vi "QTMTask.vi"(5 "timeout ms (25000)":i32=25000, 6 "Stop":bool, 7 "error in":errorcluster, 8 "ArrayIn":dbl[](array[numeric]), 9 "QTMqueue":refnum<queue>, 10 "connection ID":refnum<k5>) -> (0 "error out":errorcluster, 3 "connection ID out":refnum<k5>)   [LabVIEW 2010]
panel:
  out "ArrayOut":dbl[](array[numeric])
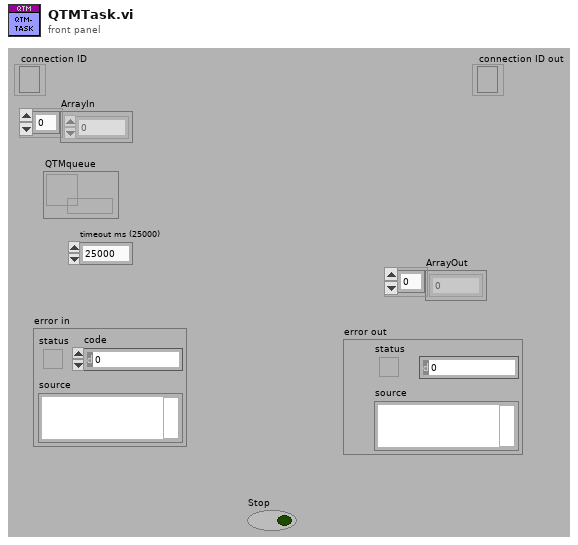
[diagram p1: front panel]
types:
  T1 = typedef "QTM Data Frame.ctl" = cluster{"Timestamp":i64, "Framenumber":i32, "ComponentCount":i32, "Components":cluster{"ComponentSize":i32, "ComponentType":T2, "Count":i32, "Padding":i32, "Data":dbl[][]}[]}
  T2 = typedef "QTM ComonentType.ctl" = i32
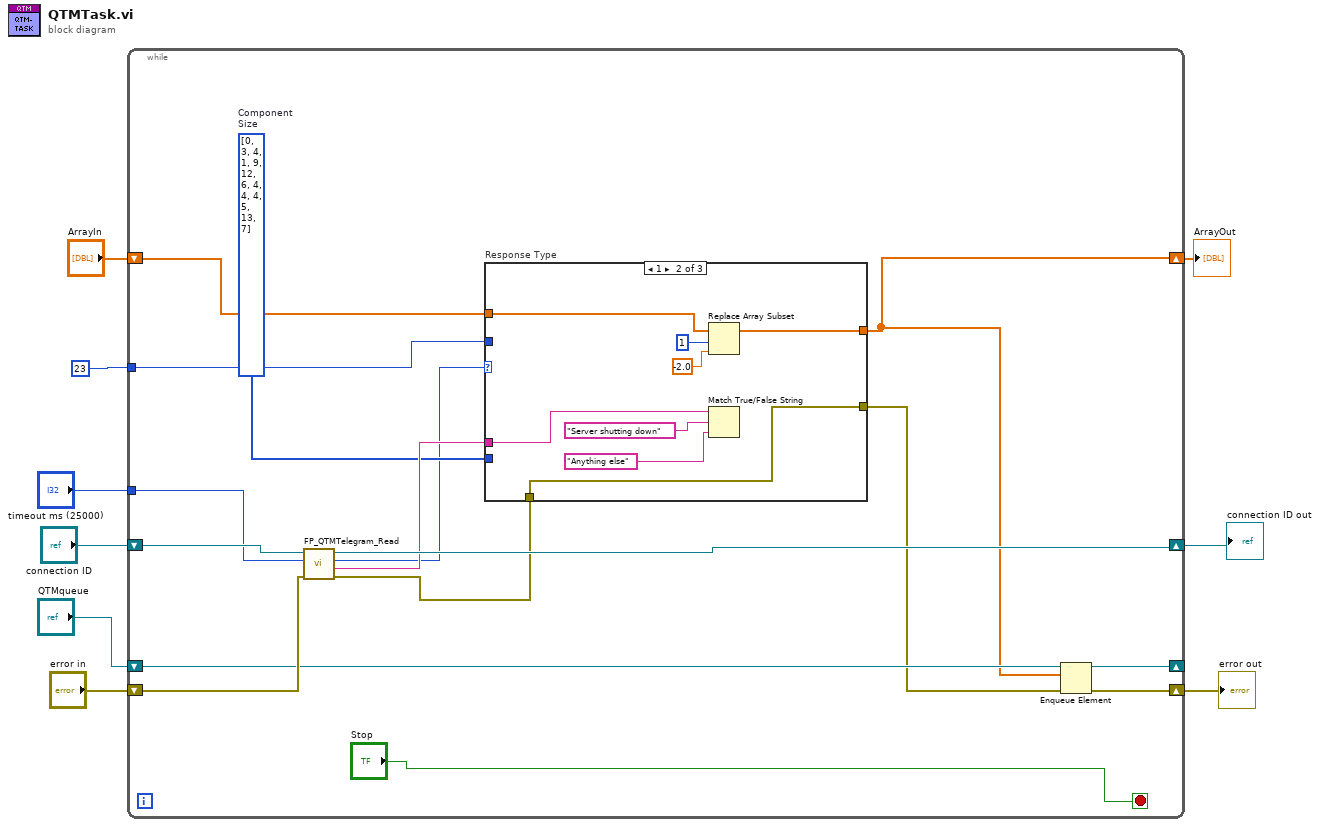
[diagram p0: block diagram]
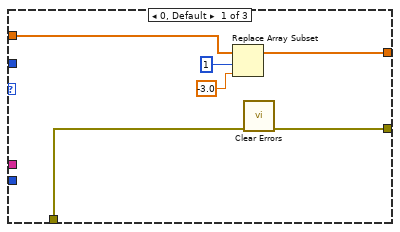
[diagram p2: hidden frame]
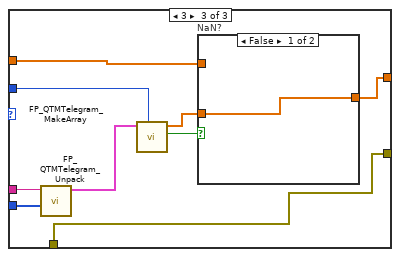
[diagram p3: hidden frame]
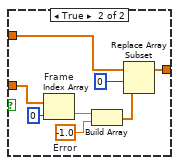
[diagram p4: hidden frame]
diagram:
  n1 = while {
    shift-right: [w12] -> w4
    shift-left: "ArrayIn" -> [w25]
    tunnel: 23 -> [w24]
    shift-right: [w13] -> w8
    shift-left: "error in" -> [w23]
    shift-right: [w21] -> w6
    shift-left: "connection ID" -> [w22]
    tunnel: "timeout ms (25000)" -> [w20]
    shift-right: [w15] -> _
    shift-left: "QTMqueue" -> [w16]
    stop <- "Stop" stop-if-true
    w18 = i32[] [0, 3, 4, 1, 9, 12, 6, 4, 4, 4, 5, 13, 7]  # Component Size
    n2 = call "FP_QTMTelegram_Read.vi"("error in (no error)"=w23, "timeout ms (25000)"=w20, "connection ID in"=w22) -> ("error out"=w14:errorcluster, "Data"=w19:string, "Response type"=w17:i32, "connection ID out"=w21:refnum<k5>)  [unwired: 5 out]
    n3 = case "Response Type" shown="1" w17 {
      tunnel: w19 -> [_ w37 w48]
      tunnel: [w30 w34 w45] -> w12
      tunnel: w18 -> [_ _ w43]
      tunnel: w24 -> [_ _ w42]
      tunnel: w25 -> [w28 w33 w41]
      tunnel: w14 -> [w27 w32 w40]
      tunnel: [w26 w32 w40] -> w10
      frame 0, Default {
        n4 = Replace Array Subset(array=w28, new element=sgl -3.0 ("new element/subarray"), index=1) -> (w30:dbl[])
        n5 = call <vilib>:"Clear Errors.vi"("error in (no error)"=w27) -> ("error out"=w26:errorcluster)  [unwired: 6 in]
      }
      frame 1 {
        n6 = Replace Array Subset(array=w33, new element=sgl -2.0 ("new element/subarray"), index=1) -> (w34:dbl[])
        n7 = Match True/False String(2:"Anything else" ("false string"), 3:"Server shutting down" ("true string"), 4:w37) -> ()  [unwired: 2 out]
      }
      frame 3 {
        n8 = call "FP_QTMTelegram_Unpack.vi"("Component\nSize"=w43, "6DOF telegram"=w48) -> ("Data Frame"=w44:T1)  [unwired: 9 out]
        n9 = call "FP_QTMTelegram_MakeArray.vi"("Array\nSize"=w42, "Data Frame"=w44) -> ("NaN?"=w47:bool, "ArrayOut"=w46:dbl[])  [unwired: 8 out]
        n10 = case "NaN?" shown="False" w47 {
          tunnel: w46 -> [w49 w55]
          tunnel: [w49 w56] -> w45
          tunnel: w41 -> [_ w50]
          frame False {
          }
          frame True {
            w52 = sgl -1.0  # Error
            n11 = Index Array "Frame"(array=w55, index=0) -> (element=w53:dbl)
            n12 = Build Array(w53, w52) -> (w51:dbl[])
            n13 = Replace Array Subset(array=w50, new element=w51, index=0) -> (w56:dbl[])
          }
        }
      }
    }
    n14 = Enqueue Element(queue=w16, element=w12, error in (no error)=w10) -> (queue out=w15:refnum<queue>, error out=w13:errorcluster)  [unwired: 1 in, 1 out]
  }
  "error out" <- w8
  "connection ID out" <- w6
  "ArrayOut" <- w4
